vi "add_agent.vi"(0 "Host_Reference":refnum<class "HGF_Reference.lvclass">, 2 "timeout in ms (-1)":i32, 3 "MoAgSy_Message":refnum<class "MoAgSy_Message.lvclass">, 5 "error in (no error)":errorcluster) -> (14 "dup Host_Reference":refnum<class "HGF_Reference.lvclass">, 16 "dup timeout in ms (-1)":i32, 19 "error out":errorcluster)   [LabVIEW 2009, in "MoAgSy.lvlib" / "MoAgSy_Host.lvclass"]
uses:
  MoAgSy_Host.lvclass
  MoAgSy_Message/MoAgSy_Message.lvclass
  HGF_BaseClasses/HGF_Reference/HGF_Reference.lvclass
  MoAgSy_AgentBase/MoAgSy_AgentBase.lvclass
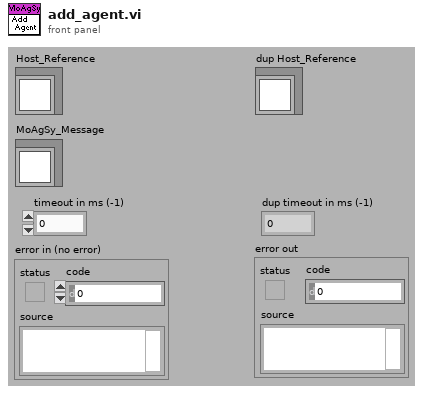
[diagram p1: front panel]
types:
  T1 = enum16{"Not a visitable", "Agent blacklisted", "Host full", "ok"}
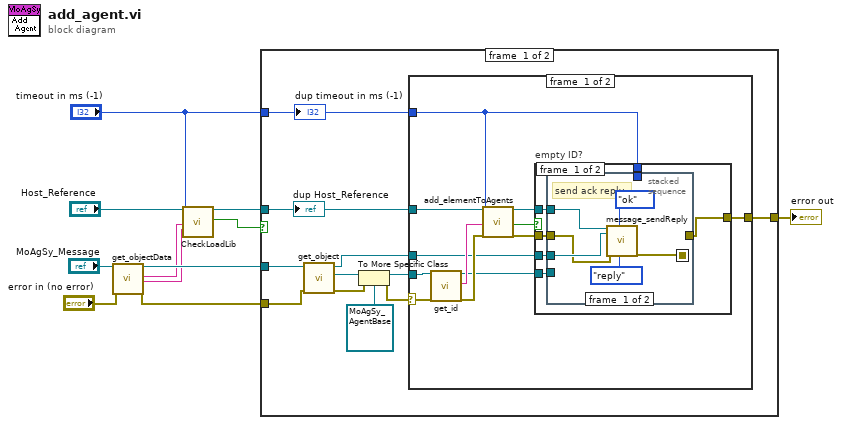
[diagram p0: block diagram]
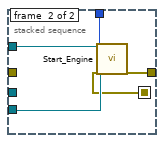
[diagram p2: hidden frame]
diagram:
  n1 = call "get_objectData.vi"("MoAgSy_Message.lvclass in"="MoAgSy_Message", "error in (no error)"="error in (no error)") -> ("MoAgSy_Message.lvclass out"=w9:refnum<class "MoAgSy_Message.lvclass">, "Object Library"=w2:string, "Object Class Name"=w1:string, "error out"=w7:errorcluster)  [unwired: 14 in]
  n2 = call "CheckLoadLib.vi"("Host_Reference"="Host_Reference", "timeout in ms (-1)"="timeout in ms (-1)", "LibraryName"=w2, "classname"=w1) -> ("dup Host_Reference"=w5:refnum<class "HGF_Reference.lvclass">, "status"=w6:bool)  [unwired: 14 in]
  n3 = case shown="False" w6 {
    tunnel: w9 -> [w22 _]
    tunnel: w7 -> [w19 w54]
    tunnel: [w16 w54] -> w11
    tunnel: "timeout in ms (-1)" -> [w14 _]
    tunnel: w5 -> [w13 _]
    frame #0 {
      n4 = call "get_object.vi"("error in (no error)"=w19, "MoAgSy_Message.lvclass in"=w22) -> ("error out"=w18:errorcluster, "Object"=w21:refnum<class>, "MoAgSy_Message.lvclass out"=w12:refnum<class "MoAgSy_Message.lvclass">)  [unwired: 7 out]
      n5 = To More Specific Class(target class=refnum<class "MoAgSy_AgentBase.lvclass"> refnum ("HGF_AgentBaseClasses.lvlib:HGF_Agent.lvclass"), reference=w21, error in=w18) -> (specific class reference=w15:refnum<class "MoAgSy_AgentBase.lvclass">, error out=w17:errorcluster)
      n6 = case shown="No Error" w17 {
        selector: w17 -> [w33 w53]
        tunnel: [w24 w53] -> w16
        tunnel: w15 -> [w34 _]
        tunnel: w14 -> [w27 _]
        tunnel: w13 -> [w32 _]
        tunnel: w12 -> [w23 _]
        frame #0 {
          n7 = call "get_id.vi"("HGF_Agent in"=w34, "error in (no error)"=w33) -> ("HGF_Agent out"=w26:refnum<class "MoAgSy_AgentBase.lvclass">, "ID"=w31:string, "error out"=w30:errorcluster)  [unwired: 15 out]
          n8 = call "add_elementToAgents.vi"("Host_Reference"=w32, "timeout in ms (-1)"=w27, "Agent ID"=w31, "error in (no error)"=w30) -> ("dup Host_Reference"=w28:refnum<class "HGF_Reference.lvclass">, "empty ID"=w29:bool, "error out"=w25:errorcluster)  [unwired: 13 out]
          n9 = case "empty ID?" shown="False" w29 {
            tunnel: w28 -> [w40 _]
            tunnel: w27 -> [w39 _]
            tunnel: w26 -> [w38 _]
            tunnel: w25 -> [w37 w52]
            tunnel: [w36 w52] -> w24
            tunnel: w23 -> [w35 _]
            frame #0 {
              n10 = stacked-sequence {
                seq-local: [w42 _] -> [_ w47]
                tunnel: w40 -> [w46 w51]
                tunnel: w39 -> [_ w50]
                tunnel: w38 -> [_ w49]
                tunnel: w37 -> [w43 _]
                tunnel: [_ w48] -> w36
                tunnel: w35 -> [w45 _]
                frame #0 {
                  # "send ack reply"
                  n11 = call "message_sendReply.vi"("Host_Reference"=w46, "MoAgSy_Message"=w45, "error in (no error)"=w43, "message"=T1."ok", "Message Type"=enum16{"error Reply", "reply", "PublicKey"}."reply") -> ("error out"=w42:errorcluster)  [unwired: 13 in, 1 out]
                }
                frame #1 {
                  n12 = call "Start_Engine.vi"("Host_Reference"=w51, "timeout in ms (-1)"=w50, "HGF_Agent"=w49, "error in (no error)"=w47) -> ("error out"=w48:errorcluster)  [unwired: 15 out]
                }
              }
            }
            frame #1 {
              # "abweisen"
            }
          }
        }
        frame #1 {
        }
      }
      "dup timeout in ms (-1)" <- w14
      "dup Host_Reference" <- w13
    }
    frame #1 {
    }
  }
  "error out" <- w11
